vi "SetCurvVisible.vi"(7 "Force vis":bool, 8 "error in (no error)":errorcluster caption="entrée d'erreur (pas d'erreur)", 10 "CurveIndex":i32, 11 "Interface en entrée":refnum<class "Interface.lvclass"> caption="DNL_LabVIEW Object in") -> (0 "error out":errorcluster caption="sortie d'erreur", 3 "Interface en sortie":refnum<class "Interface.lvclass"> caption="DNL_LabVIEW Object out")   [LabVIEW 2010, in "Interface.lvclass"]
uses:
  Interface.lvclass
  Interface.lvclass/Interface.ctl
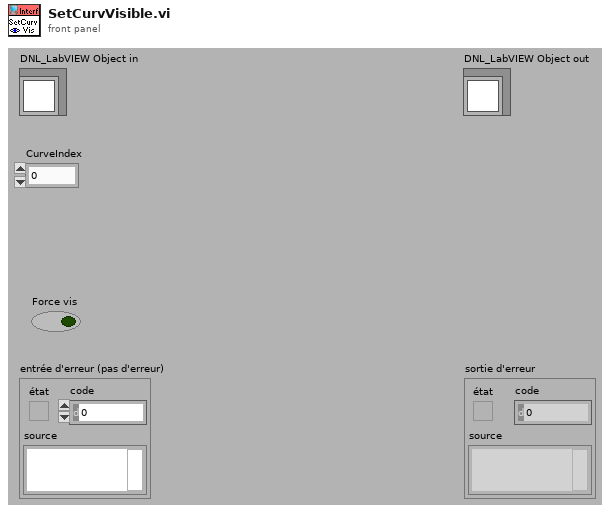
[diagram p1: front panel]
types:
  T1 = typedef "Interface.lvclass/CurveSetup.ctl" = cluster{"CurveName":string, "YParam":string, "XParam":string, "ZParam ":string, "GroupName":string, "LinWdth":u8, "PntCol":u32, "LinCol":u32, "LablFor":u8, "XScale":u32, "YScale":u32, "Interpol":u8, "DisplayName":string, "FillType":i16, "LineStyle":u8, "PntStyle":u8, "BarTyp":u8, "GraphIndex":i32, "Visible":bool, "XScaleName":string, "YScaleName":string, "XYGraph_Ref":refnum<vi>, "Data Only":bool, "DataQ Ref":refnum<queue>, "XParQ Ref":refnum<queue>, "XParamInd":i32}
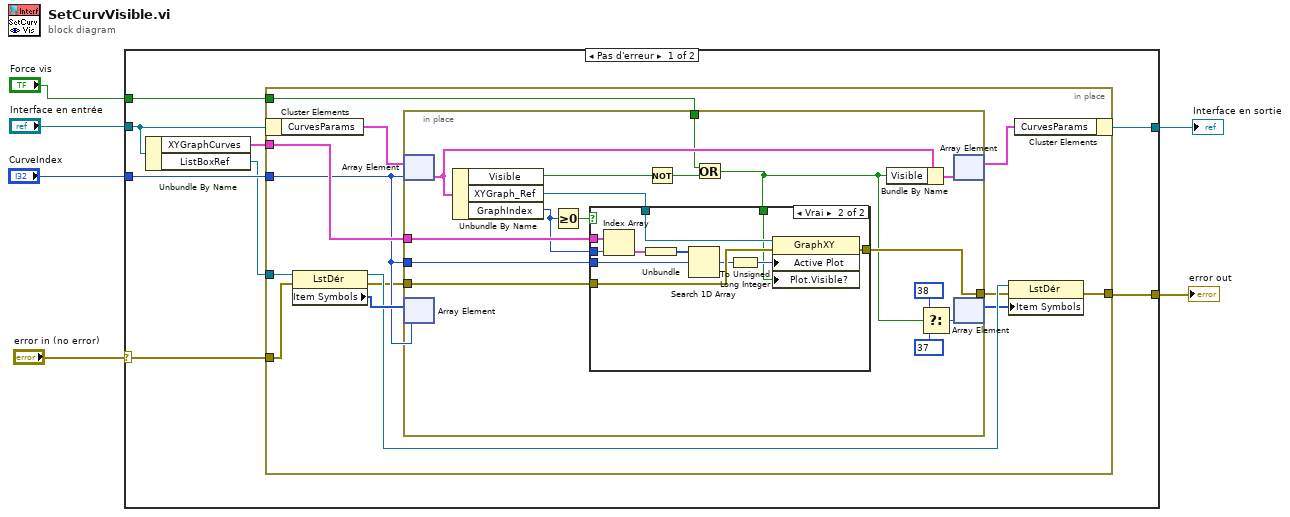
[diagram p0: block diagram]
diagram:
  n1 = case shown="Pas d'erreur" "error in (no error)" {
    selector: "error in (no error)" -> [w12 w57]
    tunnel: [w11 w57] -> w5
    tunnel: [w13 w56] -> w3
    tunnel: "Interface en entrée" -> [w10 w56]
    tunnel: "CurveIndex" -> [w14 _]
    tunnel: "Force vis" -> [w8 _]
    frame No Error {
      n2 = Unbundle By Name(w10) -> ("XYGraphCurves"=w9:cluster{"Tableau":i32[]}[], "ListBoxRef"=w7:refnum<vi>)
      n3 = in-place {
        in-place-border: w14 -> [w19]
        in-place-border: w7 -> [w25]
        in-place-border: w12 -> [w22]
        in-place-border: [w21] -> w11
        in-place-border: w9 -> [w20]
        in-place-border: w8 -> [w17]
        n4 = in-place-cluster #1(w10) -> ("CurvesParams"=w27:T1[])
        n5 = property on="Nœud de propriété" class="LstDér"(reference=w25, error in=w22) -> (reference out=w23:refnum<vi>, error out=w18:errorcluster, "Item Symbols"=w24:i32[])
        n6 = in-place {
          in-place-border: w20 -> [w37]
          in-place-border: w19 -> [w36]
          in-place-border: w18 -> [w35]
          in-place-border: w17 -> [w32]
          in-place-border: [w31] -> w16
          n7 = in-place-array #2(w27, w19) -> (w42:T1)
          n8 = in-place-array #3(w24, w19) -> ()  [unwired: 1 out]
          n9 = Unbundle By Name(w42) -> ("Visible"=w38:bool, "XYGraph_Ref"=w34:refnum<vi>, "GraphIndex"=w28:i32)
          n10 = Greater Or Equal To 0?(x=w28) -> (x >= 0?=w29:bool)
          n11 = Not(x=w38) -> (.not. x?=w33:bool)
          n12 = Or(x=w32, y=w33) -> (x .or. y?=w30:bool)
          n13 = case shown="Vrai" w29 {
            tunnel: w37 -> [_ w55]
            tunnel: w28 -> [_ w54]
            tunnel: w36 -> [_ w51]
            tunnel: w35 -> [w44 w50]
            tunnel: w34 -> [_ w47]
            tunnel: w30 -> [_ w46]
            tunnel: [w44 w45] -> w31
            frame False {
            }
            frame True {
              n14 = Index Array(array=w55, index=w54) -> (element=w53:cluster{"Tableau":i32[]})
              n15 = Unbundle(w53) -> ("Tableau"=w52:i32[])
              n16 = Search 1D Array(1D array=w52, element=w51) -> (index of element=w49:i32)  [unwired: 1 in]
              n17 = To Unsigned Long Integer(number=w49) -> (unsigned 32bit integer=w48:u32)
              n18 = property class="GraphXY"(reference=w47, error in=w50, "Active Plot"=w48, "Plot.Visible?"=w46) -> (error out=w45:errorcluster)  [unwired: 1 out]
            }
          }
          n19 = Bundle By Name(cluster=w42, "Visible"=w30) -> (w43:T1)
          n20 = Select(t=38, s=w30, f=37) -> (s? t:f=w39:i32)
          n21 = in-place-array #2(w43) -> (w26:T1[])  [unwired: 1 out]
          n22 = in-place-array #3(w39) -> (w15:i32[])  [unwired: 1 out]
        }
        n23 = property on="Nœud de propriété" class="LstDér"(reference=w23, error in=w16, "Item Symbols"=w15) -> (error out=w21:errorcluster)  [unwired: 1 out]
        n24 = in-place-cluster #1("CurvesParams"=w26) -> (w13:refnum<class "Interface.lvclass">)
      }
    }
    frame Error {
    }
  }
  "error out" <- w5
  "Interface en sortie" <- w3
